vi "Log Data.vi"(7 "Image Array (in)":T1[](array[typedef]), 8 "Error In":errorcluster, 9 "Imaging Mode":T2(ring), 10 "Data Queue":T3, 11 "Logging Configuration":T4) -> (0 "Error Out":errorcluster)   [LabVIEW 2020]
doc: "Use the Write To Measurement File Express VI to log data to disk in a LVM file."
uses:
  Typedefs/Logging Configuration.ctl
  Acquisition/Typedefs/Data queue ref.ctl
  Typedefs/Logging queue element.ctl
  Typedefs/Imaging Protocols enum.ctl
  Typedefs/Frame Size.ctl
  Typedefs/Acquired points count.ctl
  <vilib>/vision/Image Controls.llb/IMAQ Image.ctl
panel:
  in  "dwelltme(us)":dbl
  in  "Frame Size":u32
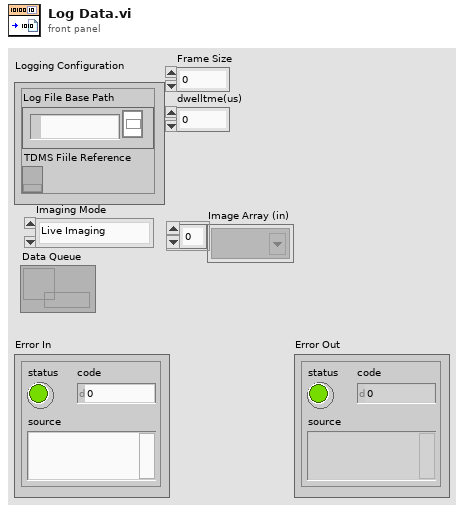
[diagram p1: front panel]
types:
  T1 = typedef "IMAQ Image.ctl" = refnum<image>
  T2 = enum16{"Live Imaging", "AOL Z Stack ", "Motor Z Stack", "Functional Imaging"}
  T3 = typedef "Data queue ref.ctl" = refnum<queue>
  T4 = typedef "Logging Configuration.ctl" = cluster{"Log File Base Path":path, "TDMS Fiile Reference":refnum<k34>}
  T5 = typedef "Logging queue element.ctl" = cluster{"Imaging Protocol":T6, "Number of Trials":u16, "Frame Size":T7, "# Averaged frames":u16, "Dwell time (us)":dbl, "Index of Z-plane":i32, "Timelapse?":bool, "Logging process is active":bool, "Speed logging enabled":bool, "tdms file ref":refnum<k34>, "path":path, "Trial Number":i32, "Expected # points acquired":bool, "Manually stopped":bool, "Last trial":bool, "Ch0 data":u32[], "Ch1 data":u32[], "Ref Data":u32[], "Ref Frame Time":u64[], "Image Time":u64[], "Continuous Time":u64[], "Ref X Length":u16, "Ref Y Length":u16, "# Ref Averaged frames":u16, "Ref Dwell time (us)":dbl, "Points acquired":T8, "HW Timings File":refnum<file>}
  T6 = typedef "Imaging Protocols enum.ctl" = enum16{"AOL Z-Stack", "Motor Z Stack", "Functional Acquisition", "Single Plane Acquisition", "Volume Acquisition", "Live Imaging", "Live Plane Imaging", "Live Volume Imaging"}
  T7 = typedef "Frame Size.ctl" = u16
  T8 = typedef "Acquired points count.ctl" = cluster{"Ch0 last trial":u64, "Ch1 last trial":u64, "All trials":u64}
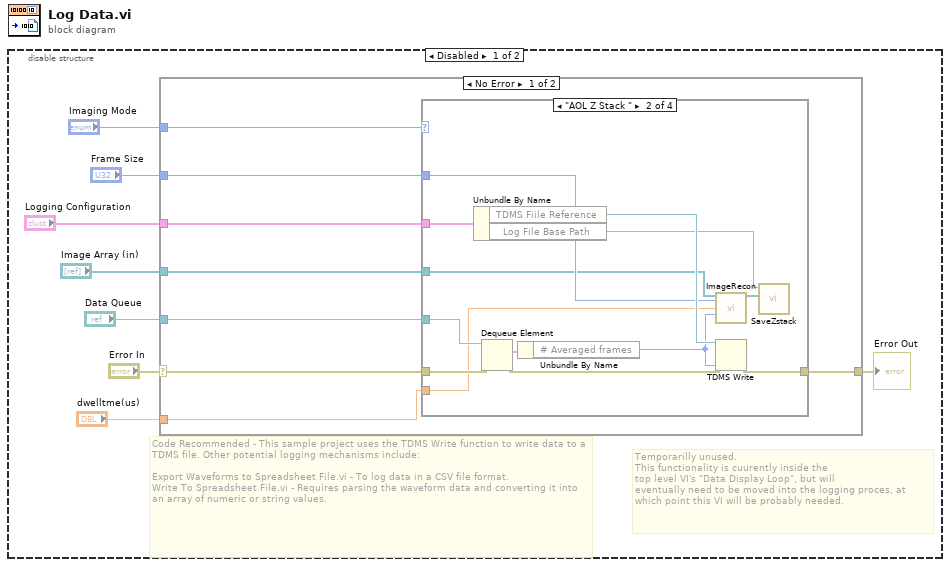
[diagram p0: block diagram]
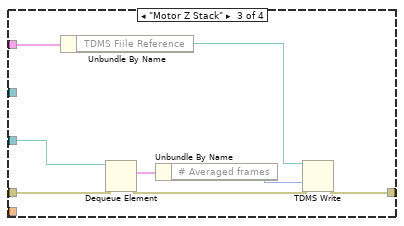
[diagram p3: hidden frame]
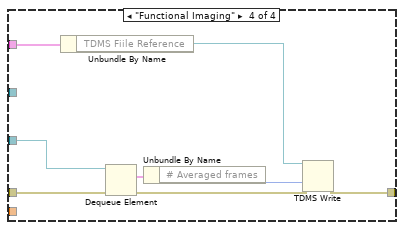
[diagram p4: hidden frame]
diagram:
  n1 = disable-structure shown="Disabled" {
    frame Disabled {
      # "Temporarilly unused.\nThis functionality is cuurently inside the\ntop level VI's \"Data Display Loop\", but will\neventually need to be moved into the logging proces, at which point this VI will be probably needed."
      # "Code Recommended - This sample project uses the TDMS Write function to write data to a TDMS file. Other potential logging mechanisms include:\n\nExport Waveforms to Spreadsheet File.vi - To log data in a CSV file format.\nWrite To Spreadsheet File.vi - Requires parsing the waveform data and converting it into an array of numeric or string values."
      n2 = case shown="No Error" "Error In" {
        selector: "Error In" -> [w15 w47]
        tunnel: "Logging Configuration" -> [w16 _]
        tunnel: "Data Queue" -> [w14 _]
        tunnel: [w13 w47] -> w5
        tunnel: "Imaging Mode" -> [w12 _]
        tunnel: "Frame Size" -> [w11 _]
        tunnel: "dwelltme(us)" -> [w10 _]
        tunnel: "Image Array (in)" -> [w9 _]
        frame No Error {
          n3 = case shown="\"AOL Z Stack \"" w12 {
            tunnel: w16 -> [_ w30 w38 w46]
            tunnel: w15 -> [w17 w29 w37 w45]
            tunnel: w14 -> [_ w28 w36 w44]
            tunnel: [w17 w26 w34 w42] -> w13
            tunnel: w11 -> [_ w23 _ _]
            tunnel: w10 -> [_ w24 _ _]
            tunnel: w9 -> [_ w20 _ _]
            frame "Live Imaging", Default {
            }
            frame "AOL Z Stack " {
              n4 = Unbundle By Name(w30) -> ("TDMS Fiile Reference"=w27:refnum<k34>, "Log File Base Path"=w22:path)
              n5 = Dequeue Element(queue=w28, error in (no error)=w29) -> (element=w19:T5, error out=w25:errorcluster)  [unwired: 1 in, 2 out]
              n6 = Unbundle By Name(w19) -> ("# Averaged frames"=w18:u16)
              n7 = call "ImageRecon.vi"("Image Array (in)"=w20, 1:w23, "dwelltime"=w24, "Waveforms"=w18) -> ("Image Array(out)"=w21:T1[])  [unwired: 8 in, 3 out]
              n8 = TDMS Write(0:w27, 9:w18, 11:w25) -> (15:w26:errorcluster)  [unwired: 3 in, 3 out]
              n9 = call "SaveZstack.vi"("ImageArray"=w21, "base path"=w22) -> ()  [unwired: 10 in]
            }
            frame "Motor Z Stack" {
              n10 = Unbundle By Name(w38) -> ("TDMS Fiile Reference"=w35:refnum<k34>)
              n11 = Dequeue Element(queue=w36, error in (no error)=w37) -> (element=w31:T5, error out=w33:errorcluster)  [unwired: 1 in, 2 out]
              n12 = Unbundle By Name(w31) -> ("# Averaged frames"=w32:u16)
              n13 = TDMS Write(0:w35, 9:w32, 11:w33) -> (15:w34:errorcluster)  [unwired: 3 in, 3 out]
            }
            frame "Functional Imaging" {
              n14 = Unbundle By Name(w46) -> ("TDMS Fiile Reference"=w43:refnum<k34>)
              n15 = Dequeue Element(queue=w44, error in (no error)=w45) -> (element=w40:T5, error out=w41:errorcluster)  [unwired: 1 in, 2 out]
              n16 = Unbundle By Name(w40) -> ("# Averaged frames"=w39:u16)
              n17 = TDMS Write(0:w43, 9:w39, 11:w41) -> (15:w42:errorcluster)  [unwired: 3 in, 3 out]
            }
          }
        }
        frame Error {
        }
      }
      "Error Out" <- w5
    }
    frame Enabled {
    }
  }
